vi "PROXY_check_database_connection.vi"(8 "error_in":errorcluster, 11 "all_config_info_in":T1) -> (0 "error_out":errorcluster, 3 "all_config_info_out":T1)   [LabVIEW 2020]
uses:
  typedef/PROXY_all_config_info.ctl
  typedef/PROXY_main_ini_file.ctl
  queues/typedef/PROXY_queue_refnums.ctl
  queues/typedef/STATION_queue_element.ctl
  STATION/ST_SQL_sequence_state.ctl
  <vilib>/addons/database/Connection.llb/DB Tools Open Connec (String).vi
  <vilib>/addons/database/NI_Database_API.lvlib
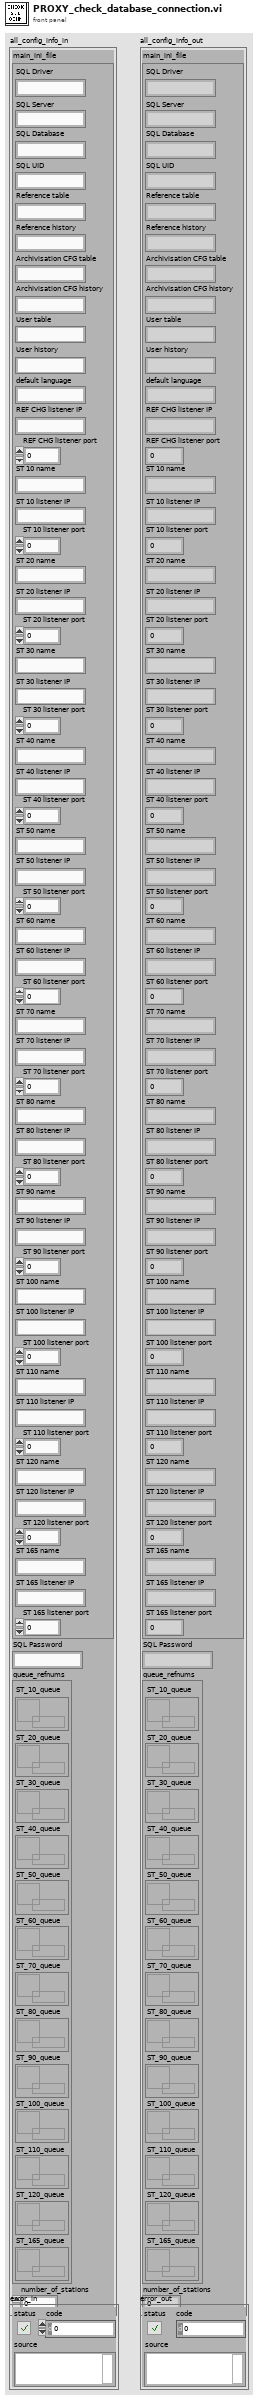
[diagram p1: front panel]
types:
  T1 = typedef "PROXY_all_config_info.ctl" = cluster{"main_ini_file":T2, "SQL Password":string, "queue_refnums":T3, "number_of_stations":i32}
  T2 = typedef "PROXY_main_ini_file.ctl" = cluster{"SQL Driver":string, "SQL Server":string, "SQL Database":string, "SQL UID":string, "Reference table":string, "Reference history":string, "Archivisation CFG table":string, "Archivisation CFG history":string, "User table":string, "User history":string, "default language":string, "REF CHG listener IP":string, "REF CHG listener port":u16, "ST 10 name":string, "ST 10 listener IP":string, "ST 10 listener port":u16, "ST 20 name":string, "ST 20 listener IP":string, "ST 20 listener port":u16, "ST 30 name":string, "ST 30 listener IP":string, "ST 30 listener port":u16, "ST 40 name":string, "ST 40 listener IP":string, "ST 40 listener port":u16, "ST 50 name":string, "ST 50 listener IP":string, "ST 50 listener port":u16, "ST 60 name":string, "ST 60 listener IP":string, "ST 60 listener port":u16, "ST 70 name":string, "ST 70 listener IP":string, "ST 70 listener port":u16, "ST 80 name":string, "ST 80 listener IP":string, "ST 80 listener port":u16, "ST 90 name":string, "ST 90 listener IP":string, "ST 90 listener port":u16, "ST 100 name":string, "ST 100 listener IP":string, "ST 100 listener port":u16, "ST 110 name":string, "ST 110 listener IP":string, "ST 110 listener port":u16, "ST 120 name":string, "ST 120 listener IP":string, "ST 120 listener port":u16, "ST 165 name":string, "ST 165 listener IP":string, "ST 165 listener port":u16}
  T3 = typedef "PROXY_queue_refnums.ctl" = cluster{"ST_10_queue":refnum<queue>, "ST_20_queue":refnum<queue>, "ST_30_queue":refnum<queue>, "ST_40_queue":refnum<queue>, "ST_50_queue":refnum<queue>, "ST_60_queue":refnum<queue>, "ST_70_queue":refnum<queue>, "ST_80_queue":refnum<queue>, "ST_90_queue":refnum<queue>, "ST_100_queue":refnum<queue>, "ST_110_queue":refnum<queue>, "ST_120_queue":refnum<queue>, "ST_165_queue":refnum<queue>}
  T4 = typedef "NI_Database_API.lvlib/Conn ObjectReference.ctl" = refnum<k1>
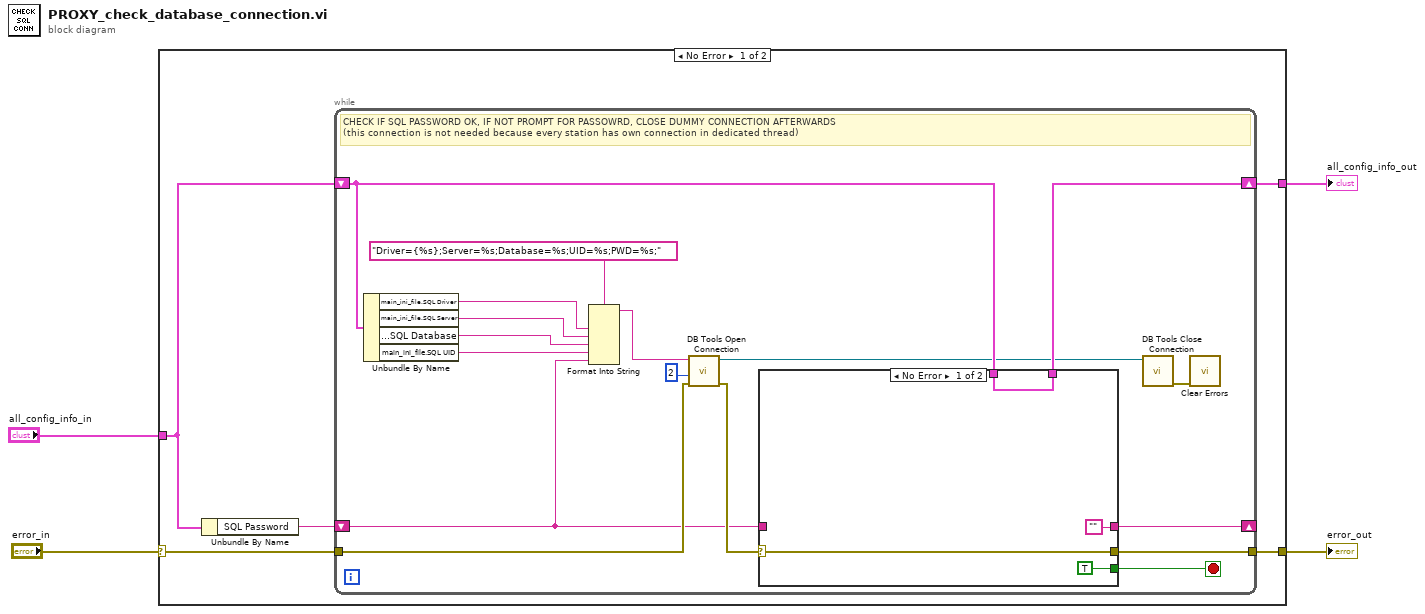
[diagram p0: block diagram]
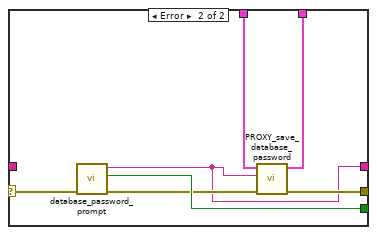
[diagram p2: hidden frame]
diagram:
  n1 = case shown="No Error" "error_in" {
    selector: "error_in" -> [w9 w38]
    tunnel: [w8 w38] -> w2
    tunnel: [w7 w39] -> w3
    tunnel: "all_config_info_in" -> [w5 w39]
    frame No Error {
      n2 = Unbundle By Name(w5) -> ("SQL Password"=w6:string)
      n3 = while {
        shift-right: [w15] -> _
        shift-left: w6 -> [w16]
        tunnel: w9 -> [w20]
        tunnel: [w14] -> w8
        shift-right: [w13] -> w7
        shift-left: w5 -> [w12]
        stop <- w18 stop-if-true
        # "CHECK IF SQL PASSWORD OK, IF NOT PROMPT FOR PASSOWRD, CLOSE DUMMY CONNECTION AFTERWARDS\n(this connection is not needed because every station has own connection in dedicated thread)"
        n4 = Unbundle By Name(w12) -> ("main_ini_file.SQL Driver"=w24:string, "main_ini_file.SQL Server"=w23:string, "main_ini_file.SQL Database"=w22:string, "main_ini_file.SQL UID"=w17:string)
        n5 = Format Into String(format string="Driver={%s};Server=%s;Database=%s;UID=%s;PWD=%s;", w24, w23, w22, w17, w16) -> (resulting string=w26:string)  [unwired: 2 in, 1 out]
        n6 = call-poly <vilib>:"DB Tools Open Connection.vi"("error in (no error)"=w20, "connection timeout (15)"=2, "connection information"=w26) -> ("error out"=w19:errorcluster, "connection reference"=w11:T4)  [unwired: 5 in]
        n7 = case shown="No Error" w19 {
          selector: w19 -> [w30 w37]
          tunnel: [w30 w32] -> w14
          tunnel: [TRUE w36] -> w18
          tunnel: w16 -> [_ _]
          tunnel: w12 -> [w28 w34]
          tunnel: [w28 w33] -> w13
          tunnel: ["" w31] -> w15
          frame No Error {
          }
          frame Error {
            n8 = call "database_password_prompt.vi"("error_in"=w37) -> ("error_out"=w35:errorcluster, "Canceled?"=w36:bool, "new_password"=w31:string)  [unwired: 8 in]
            n9 = call "PROXY_save_database_password.vi"("error_in"=w35, "new_password"=w31, "all_config_info_in"=w34) -> ("error_out"=w32:errorcluster, "all_config_info_out"=w33:T1)  [unwired: 6 in]
          }
        }
        n10 = call <vilib>:"DB Tools Close Connection.vi"("connection reference"=w11) -> ("error out"=w10:errorcluster)  [unwired: 6 in]
        n11 = call <vilib>:"Clear Errors.vi"("error in (no error)"=w10) -> ()  [unwired: 5 in, 2 out]
      }
    }
    frame Error {
    }
  }
  "all_config_info_out" <- w3
  "error_out" <- w2
